vi "Create GUI Element.vi"(8 "error in (no error)":errorcluster, 11 "Schedule Cell in":refnum<class "Schedule Cell.lvclass">) -> (0 "error out":errorcluster, 2 "RUN properties":T1={"Background Color"=16777226, "Number of cycles"=1, "Single RUN"={"Script Name"="", "Parameters"=[], "FPGA Name"=""}, "Quality check"=FALSE, "Cell Type"=""} {"Number of cycles" min=1}, 3 "Schedule Cell out":refnum<class "Schedule Cell.lvclass">)   [LabVIEW 2020, in "TALOS.lvlib" / "Run Utilities.lvlib" / "Schedule Cell.lvclass"]
doc: "Create a GUI object with information about the Schedule Cell"
uses:
  Schedule Cell.lvclass
  Cell - GUI.ctl
  Run Instance/Run Instance - GUI.ctl
  Run Instance/Run Instance.lvclass
  Schedule Cell.lvclass/Schedule Cell.ctl
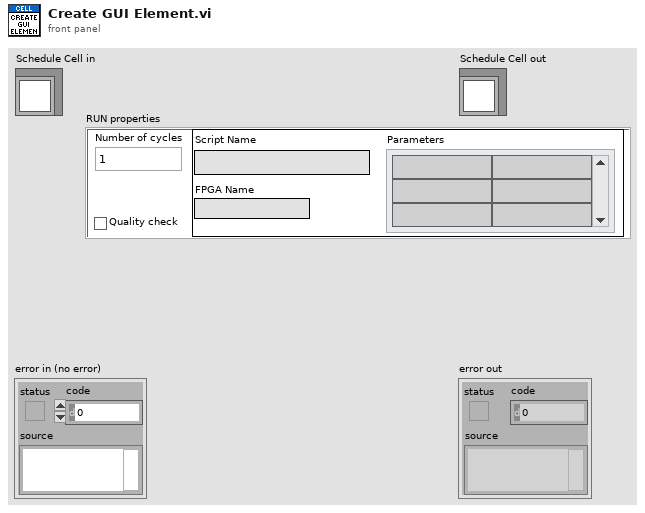
[diagram p1: front panel]
types:
  T1 = typedef "TALOS.lvlib/Run Utilities.lvlib/Schedule Cell.lvclass/Cell - GUI.ctl" = cluster{"Background Color":u32, "Number of cycles":u32, "Single RUN":T2, "Quality check":bool, "Cell Type":string}
  T2 = typedef "TALOS.lvlib/Run Utilities.lvlib/Run Instance.lvclass/Run Instance - GUI.ctl" = cluster{"Script Name":string, "Parameters":string[][], "FPGA Name":string}
  T3 = cluster{"Name":string, "Comparison":string, "Value":string}[]
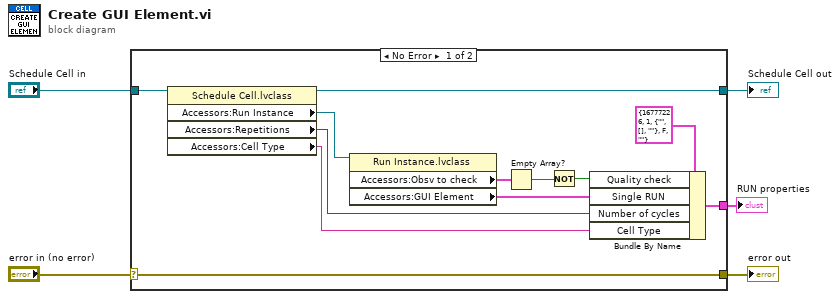
[diagram p0: block diagram]
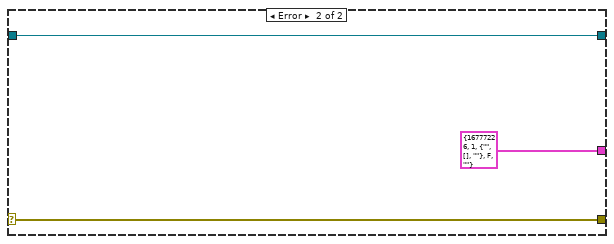
[diagram p2: hidden frame]
diagram:
  n1 = case shown="No Error" "error in (no error)" {
    selector: "error in (no error)" -> [w17 w20]
    tunnel: [w17 w20] -> w4
    tunnel: [w9 w19] -> w2
    tunnel: "Schedule Cell in" -> [w10 w19]
    tunnel: [w15 T1 {"Background Color"=16777226, "Number of cycles"=1, "Single RUN"={"Script Name"="", "Parameters"=[], "FPGA Name"=""}, "Quality check"=FALSE, "Cell Type"=""} ("RUN properties")] -> w1
    frame No Error {
      n2 = property class="Schedule Cell.lvclass"(reference=w10) -> (reference out=w9:refnum<class "Schedule Cell.lvclass">, "Accessors:Run Instance"=w8:refnum<class "Run Instance.lvclass">, "Accessors:Repetitions"=w7:u32, "Accessors:Cell Type"=w6:string)  [unwired: 1 in, 1 out]
      n3 = property class="Run Instance.lvclass"(reference=w8) -> ("Accessors:Obsv to check"=w14:T3, "Accessors:GUI Element"=w13:T2)  [unwired: 1 in, 2 out]
      n4 = Empty Array?(array=w14) -> (empty?=w12:bool)
      n5 = Not(x=w12) -> (.not. x?=w11:bool)
      n6 = Bundle By Name(cluster=T1 {"Background Color"=16777226, "Number of cycles"=1, "Single RUN"={"Script Name"="", "Parameters"=[], "FPGA Name"=""}, "Quality check"=FALSE, "Cell Type"=""} ("RUN properties"), "Quality check"=w11, "Single RUN"=w13, "Number of cycles"=w7, "Cell Type"=w6) -> (w15:T1)
    }
    frame Error {
    }
  }
  "error out" <- w4
  "Schedule Cell out" <- w2
  "RUN properties" <- w1
